vi "create_component_class.vi"(7 "component name":string, 8 "error in (no error)":errorcluster, 9 "component project folder path":path, 10 "parent component class path":path, 11 "project reference in":refnum<vi>) -> (0 "error out":errorcluster, 1 "new component template path":path, 2 "new class reference out":refnum<vi>, 3 "project reference out":refnum<vi>)   [LabVIEW 2010]
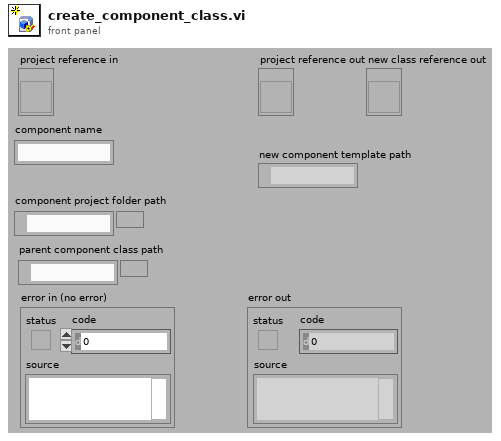
[diagram p1: front panel]
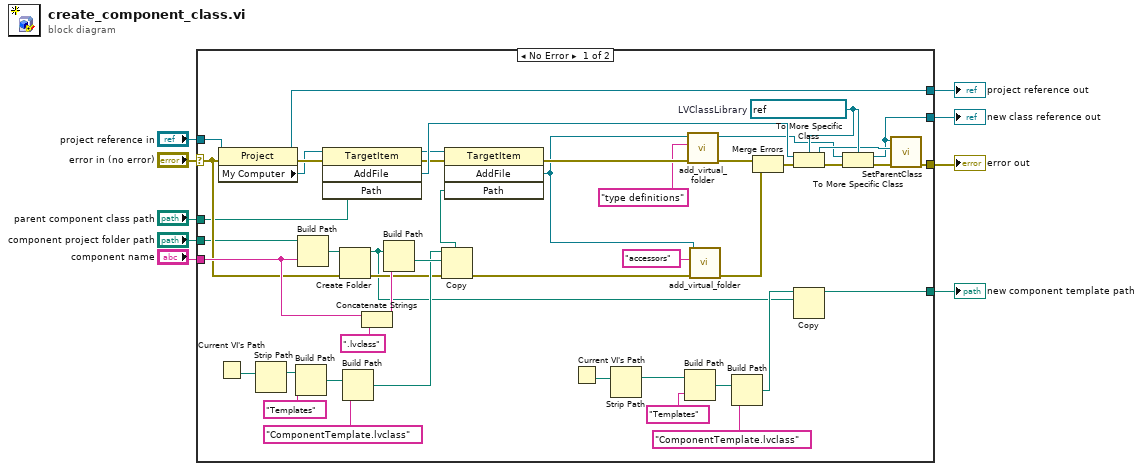
[diagram p0: block diagram]
diagram:
  n1 = case shown="No Error" "error in (no error)" {
    selector: "error in (no error)" -> [w37 w57]
    tunnel: [w45 w57] -> w9
    tunnel: "project reference in" -> [w53 w56]
    tunnel: "component name" -> [w48 _]
    tunnel: "parent component class path" -> [w36 _]
    tunnel: "component project folder path" -> [w21 _]
    tunnel: [w28 w56] -> w2
    tunnel: [w30 _] -> w3
    tunnel: [w19 _] -> w1
    frame No Error {
      w35 = refnum<vi> refnum  # LVClassLibrary
      n2 = Current VI's Path() -> (path=w44:path)
      n3 = property class="Project"(reference=w53, error in=w37) -> (reference out=w28:refnum<vi>, error out=w55:errorcluster, "My Computer"=w29:refnum<vi>)
      n4 = Strip Path(path=w44) -> (stripped path=w43:path)  [unwired: 1 out]
      n5 = Build Path(base path=w43, name or relative path="Templates") -> (appended path=w41:path)
      n6 = Build Path(base path=w21, name or relative path=w48) -> (appended path=w52:path)
      n7 = invoke on="Invoke Node" class="TargetItem" method="AddFile"(reference=w29, error in=w55, "Path"=w36) -> (reference out=w46:refnum<vi>, error out=w47:errorcluster, "AddFile"=w54:refnum<vi>)  [unwired: 1 in, 1 out]
      n8 = Create Folder(path (use dialog)=w52, error in=w37) -> (created path=w20:path, error out=w38:errorcluster)  [unwired: 1 in, 1 out]
      n9 = Build Path(base path=w41, name or relative path="ComponentTemplate.lvclass") -> (appended path=w39:path)
      n10 = Concatenate Strings(w48, ".lvclass" ("name or relative path")) -> (w50:string)
      n11 = Build Path(base path=w20, name or relative path=w50) -> (appended path=w49:path)
      n12 = Copy(8:w38, 10:w49, 11:w39) -> (0:w12:errorcluster, 3:w16:path)  [unwired: 2 in, 1 out]
      n13 = invoke on="Invoke Node" class="TargetItem" method="AddFile"(reference=w46, error in=w47, "Path"=w16) -> (error out=w18:errorcluster, "AddFile"=w13:refnum<vi>)  [unwired: 1 in, 2 out]
      n14 = Current VI's Path() -> (path=w23:path)
      n15 = Strip Path(path=w23) -> (stripped path=w24:path)  [unwired: 1 out]
      n16 = Build Path(base path=w24, name or relative path="Templates") -> (appended path=w26:path)
      n17 = call "add_virtual_folder.vi"("error in"=w18, "Name"="type definitions", "folder reference in"=w13) -> ("error out"=w17:errorcluster, "folder reference out"=w15:refnum<vi>)  [unwired: 7 in]
      n18 = call "add_virtual_folder.vi"("error in"=w12, "Name"="accessors", "folder reference in"=w13) -> ("error out"=w10:errorcluster)  [unwired: 7 in, 1 out]
      n19 = Build Path(base path=w26, name or relative path="ComponentTemplate.lvclass") -> (appended path=w22:path)
      n20 = Merge Errors(w17, w10) -> (w31:errorcluster)
      n21 = To More Specific Class(target class=w35, reference=w54, error in=w31) -> (specific class reference=w34:refnum<vi>, error out=w32:errorcluster)
      n22 = Copy(10:w20, 11:w22) -> (3:w19:path)  [unwired: 3 in, 2 out]
      n23 = To More Specific Class(target class=w35, reference=w15, error in=w32) -> (specific class reference=w30:refnum<vi>, error out=w33:errorcluster)
      n24 = call "SetParentClass.vi"("error in (no error)"=w33, "Parent Class"=w34, "LVClassLibraryRef in"=w30) -> ("error out"=w45:errorcluster)  [unwired: 7 in, 1 out]
    }
    frame Error {
    }
  }
  "error out" <- w9
  "new class reference out" <- w3
  "project reference out" <- w2
  "new component template path" <- w1
